vi "PLL.vi"(8 "error in (no error)":errorcluster, 11 "Instrument.DAQ in":refnum<class "Instrument.DAQ.lvclass">) -> (0 "error out":errorcluster, 1 "phase out":dbl, 2 "frequency out":dbl, 3 "Instrument.DAQ out":refnum<class "Instrument.DAQ.lvclass">)   [LabVIEW 2019, in "Instrument.Lockin.lvlib" / "Instrument.DAQ.lvclass"]
uses:
  Instrument.DAQ.lvclass
  Instrument.DAQ.lvclass/Instrument.DAQ.ctl
  DSP/DSP.lvclass
panel:
  in  "PLL":bool
  in  "FLL":bool
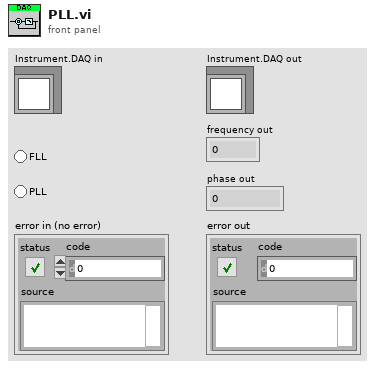
[diagram p1: front panel]
types:
  T1 = typedef "Instrument.Lockin.lvlib/Instrument.DAQ.lvclass/PublicEvents--DAQ.getWaveforms.ctl" = cluster{"AO":waveform(dbl)[], "AI":waveform(dbl)[], "REF_X":waveform(dbl)[], "REF_Y":waveform(dbl)[], "X":waveform(dbl)[], "Y":waveform(dbl)[]}
  T2 = typedef "Instrument.Lockin.lvlib/Instrument.DAQ.lvclass/AI.Channel--Cluster--Array.ctl" = T3[]
  T3 = typedef "Instrument.Lockin.lvlib/Instrument.DAQ.lvclass/AI.Channel--Cluster.ctl" = cluster{"Enable?":bool, "Channel":i32, "References":u16[], "reference index":i32}
  T4 = typedef "Instrument.Lockin.lvlib/Instrument.DAQ.lvclass/REF.Channel--Cluster--Array.ctl" = T5[]
  T5 = typedef "Instrument.Lockin.lvlib/Instrument.DAQ.lvclass/REF.Channel--Cluster.ctl" = cluster{"Enable?":bool, "Channel":i32, "Frequency":dbl, "Phase":dbl, "TC":dbl, "Roll-Off":i32}
  T6 = typedef "Instrument.Lockin.lvlib/Instrument.DAQ.lvclass/DAQ.Sampling--Cluster.ctl" = cluster{"Sampling":T7, "Fs_Out":dbl}
  T7 = typedef "Instrument.Lockin.lvlib/Instrument.DAQ.lvclass/DAQ.Sampling.Sampling--Cluster.ctl" = cluster{"Fs":dbl, "#s":i32}
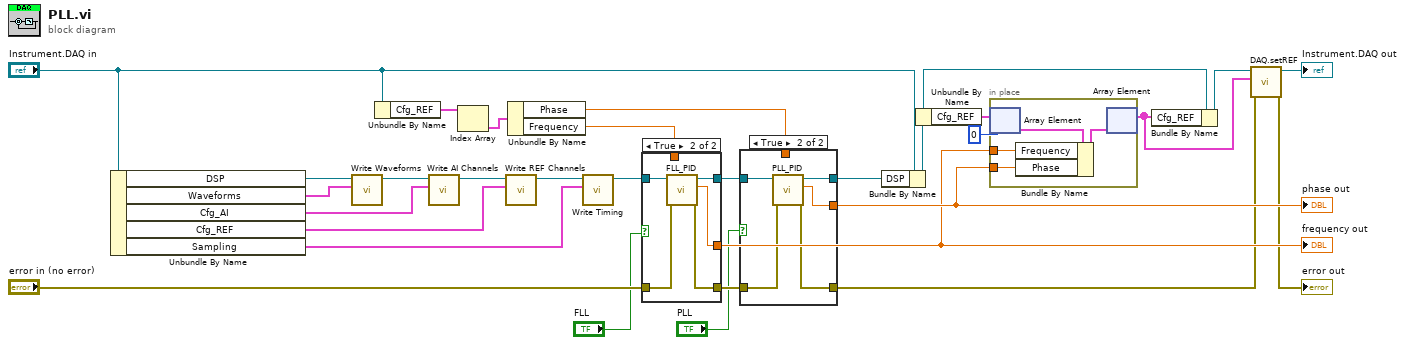
[diagram p0: block diagram]
diagram:
  n1 = Unbundle By Name("Instrument.DAQ in") -> ("DSP"=w16:refnum<class "DSP.lvclass">, "Waveforms"=w15:T1, "Cfg_AI"=w14:T2, "Cfg_REF"=w10:T4, "Sampling"=w9:T6)
  n2 = call "Write Waveforms.vi"("Waveforms"=w15, "DSP in"=w16) -> ("DSP out"=w13:refnum<class "DSP.lvclass">)  [unwired: 8 in, 1 out]
  n3 = Unbundle By Name("Instrument.DAQ in") -> ("Cfg_REF"=w4:T4)
  n4 = call "Write AI Channels.vi"("AI Channels"=w14, "DSP in"=w13) -> ("DSP out"=w12:refnum<class "DSP.lvclass">)  [unwired: 8 in, 1 out]
  n5 = Index Array(array=w4) -> (element=w3:T5)  [unwired: 1 in]
  n6 = call "Write REF Channels.vi"("REF Channels"=w10, "DSP in"=w12) -> ("DSP out"=w11:refnum<class "DSP.lvclass">)  [unwired: 8 in, 1 out]
  n7 = Unbundle By Name(w3) -> ("Phase"=w1:dbl, "Frequency"=w2:dbl)
  n8 = call "Write Timing.vi"("Timing"=w9, "DSP in"=w11) -> ("DSP out"=w8:refnum<class "DSP.lvclass">)  [unwired: 8 in, 1 out]
  n9 = case shown="True" "FLL" {
    tunnel: [w31 w38] -> w28
    tunnel: [w32 w37] -> w25
    tunnel: [w33 w36] -> w24
    tunnel: "error in (no error)" -> [w33 w35]
    tunnel: w8 -> [w32 w34]
    tunnel: w2 -> [w31 _]
    frame False {
    }
    frame True {
      n10 = call "FLL_PID.vi"("error in (no error)"=w35, "DSP.lvclass"=w34) -> ("error out"=w36:errorcluster, "frequency output (Hz)"=w38:dbl, "DSP.lvclass"=w37:refnum<class "DSP.lvclass">)  [unwired: 7 in]
    }
  }
  "frequency out" <- w28
  n11 = case shown="True" "PLL" {
    tunnel: [w39 w46] -> w29
    tunnel: [w40 w45] -> w26
    tunnel: w25 -> [w40 w44]
    tunnel: w24 -> [w41 w43]
    tunnel: [w41 w42] -> w20
    tunnel: w1 -> [w39 _]
    frame False {
    }
    frame True {
      n12 = call "PLL_PID.vi"("error in (no error)"=w43, "DSP.lvclass"=w44) -> ("error out"=w42:errorcluster, "phase out"=w46:dbl, "DSP.lvclass"=w45:refnum<class "DSP.lvclass">)  [unwired: 7 in]
    }
  }
  "phase out" <- w29
  n13 = Bundle By Name(cluster="Instrument.DAQ in", "DSP"=w26) -> (w22:refnum<class "Instrument.DAQ.lvclass">)
  n14 = Unbundle By Name(w22) -> ("Cfg_REF"=w27:T4)
  n15 = in-place {
    in-place-border: w28 -> [w48]
    in-place-border: w29 -> [w47]
    n16 = in-place-array #1(w27, 0) -> (w49:T5)
    n17 = Bundle By Name(cluster=w49, "Frequency"=w48, "Phase"=w47) -> (w50:T5)
    n18 = in-place-array #1(w50) -> (w21:T4)  [unwired: 1 out]
  }
  n19 = Bundle By Name(cluster=w22, "Cfg_REF"=w21) -> (w17:refnum<class "Instrument.DAQ.lvclass">)
  n20 = call "DAQ.setREF.vi"("error in (no error)"=w20, "Channels: Lockin"=w21, "Instrument.DAQ"=w17) -> ("error out"=→"error out":errorcluster, "Instrument.DAQ out"=→"Instrument.DAQ out":refnum<class "Instrument.DAQ.lvclass">)  [unwired: 7 in]
